vi "bats.parser.vi"(9 "data.valid":bool, 10 "data":T1={"enabled"=[FALSE, FALSE, FALSE, FALSE, FALSE, FALSE, FALSE, FALSE], "byte"=[0, 0, 0, 0, 0, 0, 0, 0]} {"byte" format="%.0x"}, 11 "reset":bool) -> (2 "Ready.for.Udp.Input":bool)   [LabVIEW 2020]
uses:
  bats.parser.state.data.ctl
  bats.parser.state.command.ctl
  <vilib>/rvi/DataTransferAndStorage/Container/XNode/niFpgaContainer.xnode
  debug/debug.type.ctl
  <vilib>/rvi/FIFO/Fifo_Resource/nirvififoEmulationWrite.vi
  data.ctl
panel:
  out "buffer.out":u64[](array[numeric]) format="%.0x"
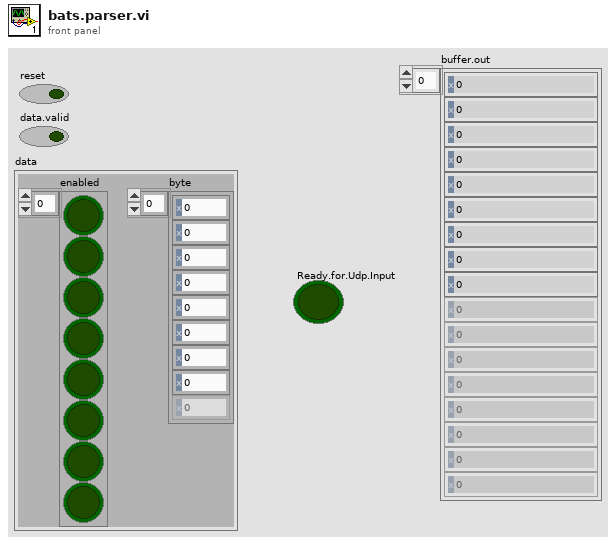
[diagram p1: front panel]
types:
  T1 = typedef "data.ctl" = cluster{"enabled":bool[], "byte":u8[]}
  T2 = typedef "bats.parser.state.command.ctl" = enum16{"Reset", "Noop", "Read.Sequenced.Unit.Header", "Read.Msg"}
  T3 = typedef "bats.parser.state.data.ctl" = cluster{"BATS.Parser.States":T2, "Saved.BATS.Parser.State":T2, "Hdr Length (U16)":u16, "MessageLength (U8)":u8, "MessageType (U8)":u8, "Time (U32)":u32, "Total Counter (U16)":u16, "Message Counter (U8)":u8, "i":u16, "Number.of.Tickers":u16, "n":u16, "msg.counter":u8, "msg.length":u8, "buffer.start":u8, "buffer.length":u8, "buffer":u64[], "Debug":T4}
  T4 = typedef "debug.type.ctl" = cluster{"Write.to.Debug":bool, "Data":u64}
  T5 = cluster{"reset":bool, "data":T1, "data.valid":bool}
  T6 = typedef "orderbook.command.ctl" = cluster{"type":T7, "side":u8, "orderId ":u64, "quantity":u32, "symbol":u64, "price":u64, "executed.qty":u32, "canceled.qty":u32, "remaining.qty":u32, "seconds":u64, "nanoseconds":u64, "Add":bool, "Edit":bool, "Remove":bool}
  T7 = typedef "orderbook.command.type.ctl" = enum8{"Time", "AddOrder", "OrderExecuted", "OrderExecutedAtPrice", "ReduceSize", "ModifyOrder", "DeleteOrder", "Get.Everything", "Get.All.Orders", "Get.Top"}
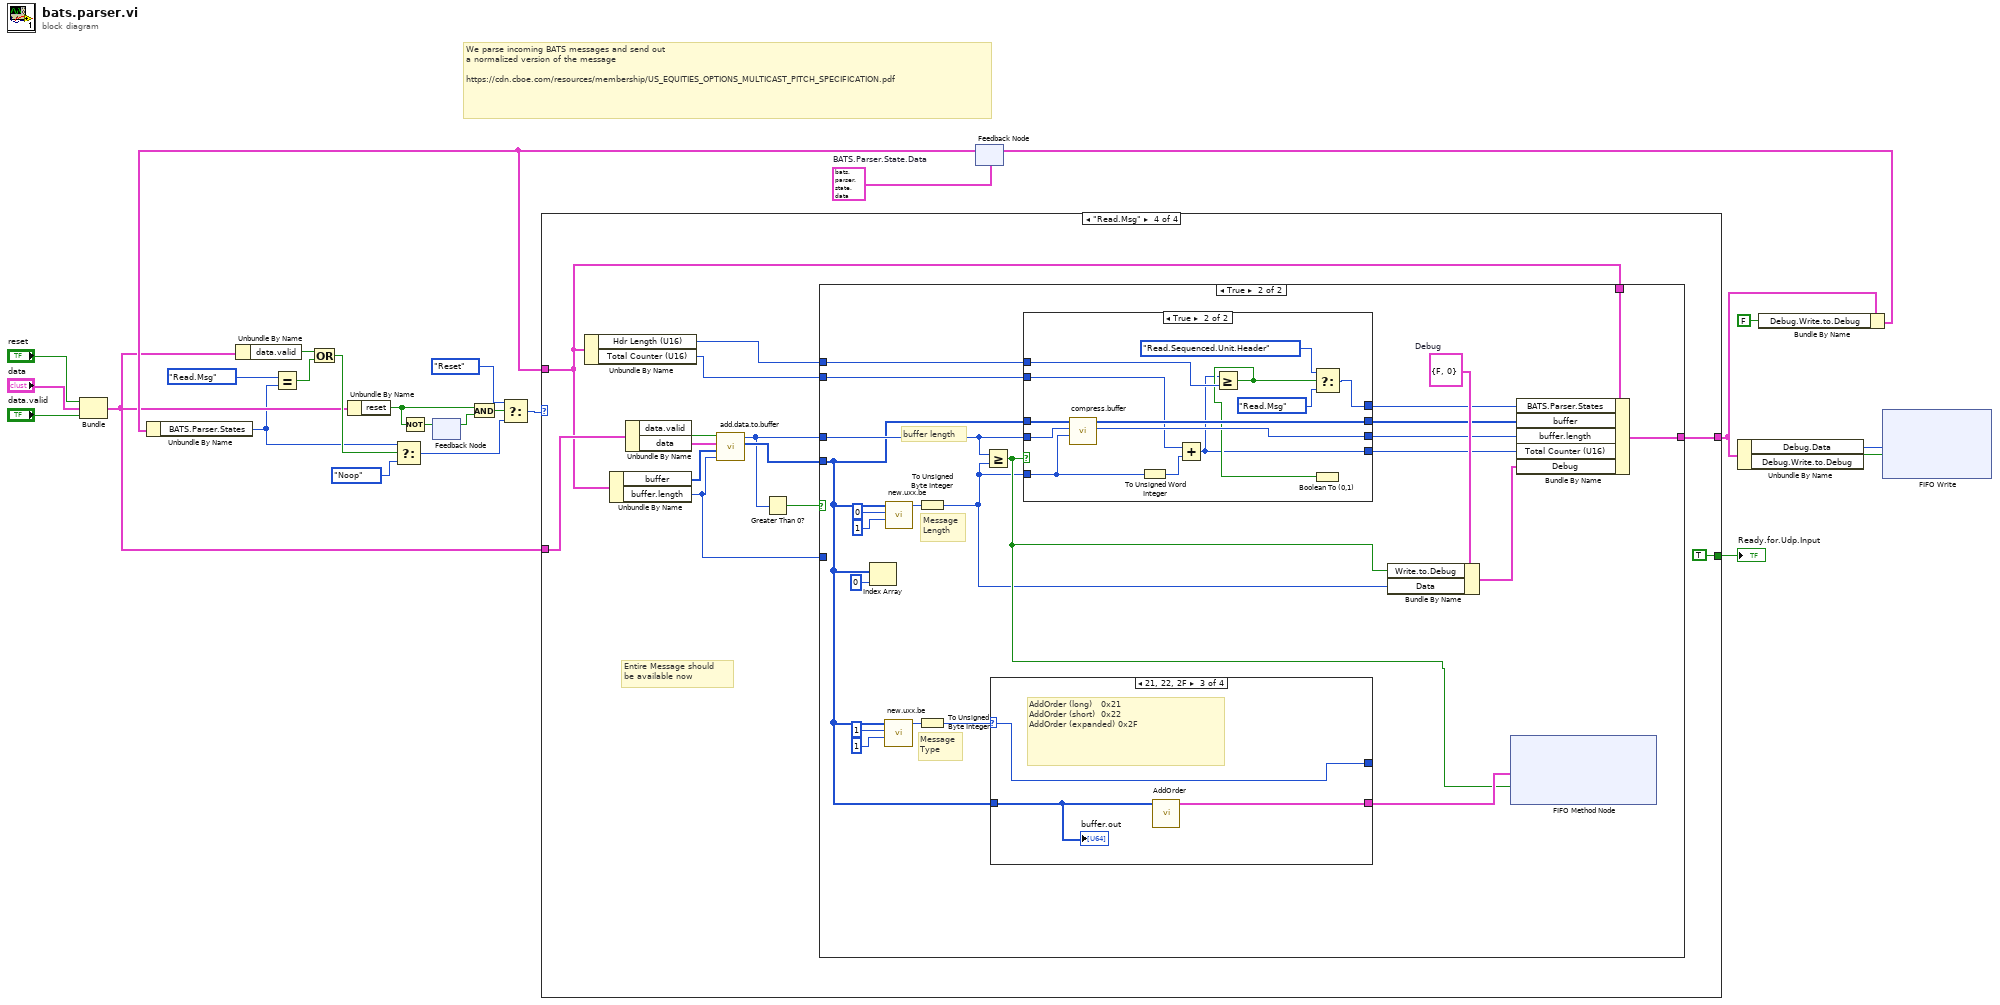
[diagram p0: block diagram]
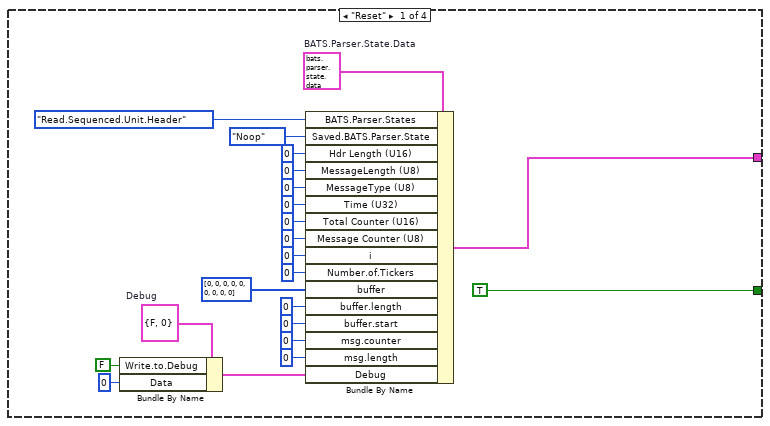
[diagram p2: hidden frame]
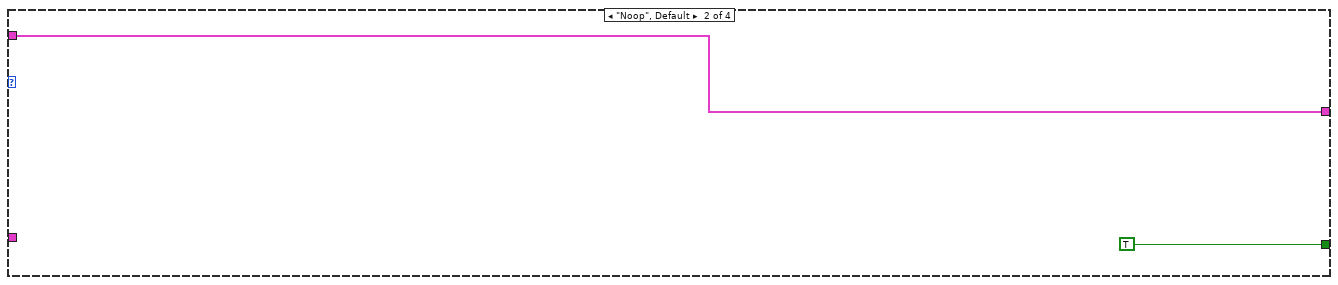
[diagram p3: hidden frame]
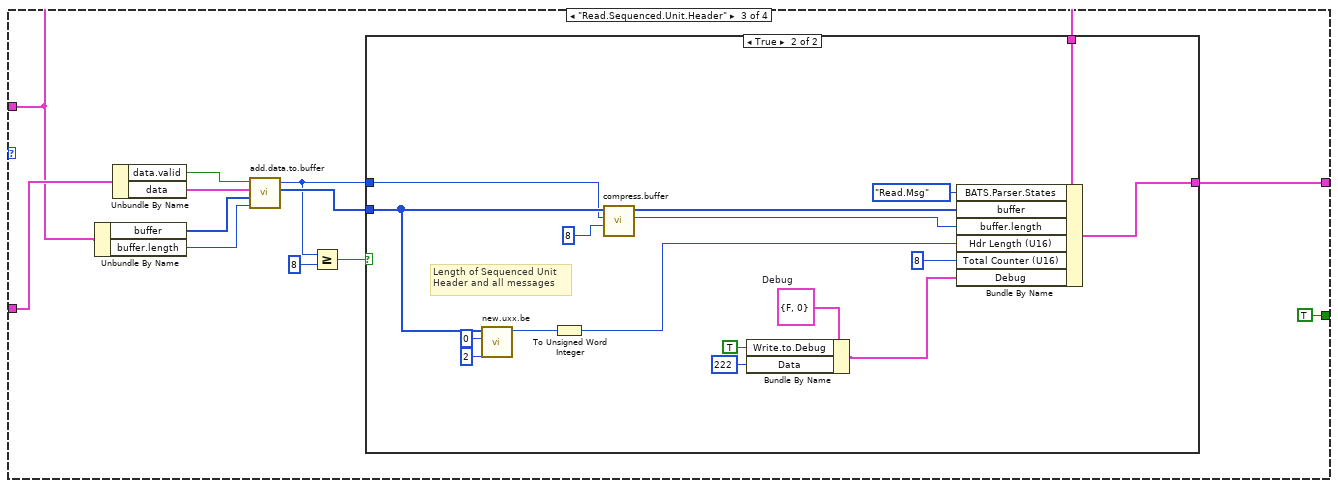
[diagram p4: hidden frame]
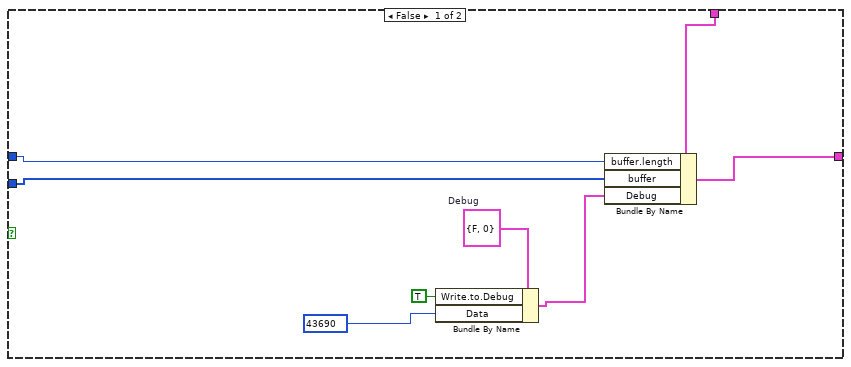
[diagram p5: hidden frame]
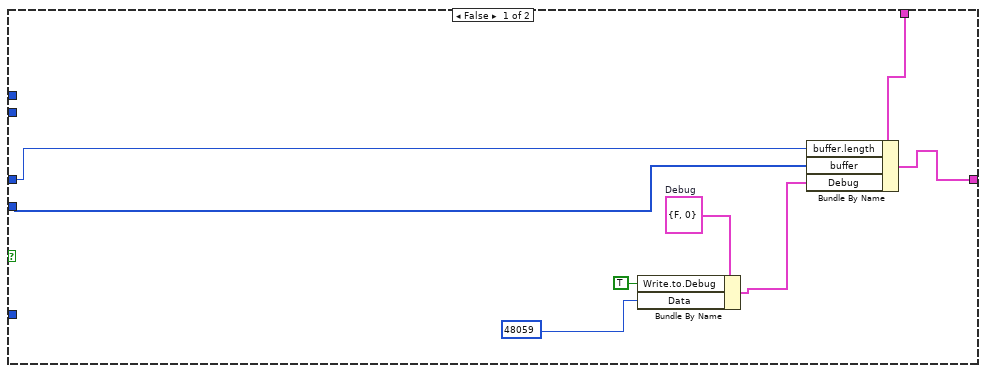
[diagram p6: hidden frame]
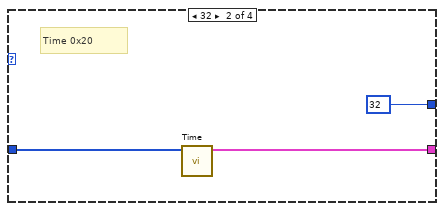
[diagram p8: hidden frame]
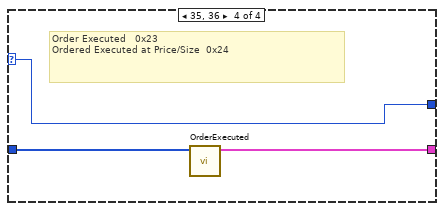
[diagram p9: hidden frame]
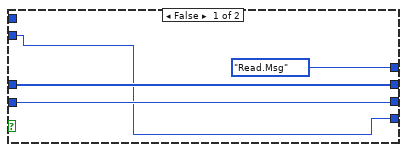
[diagram p10: hidden frame]
diagram:
  w25 = T3 {"BATS.Parser.States"=enum."Read.Sequenced.Unit.Header", "Saved.BATS.Parser.State"=enum."Reset", "Hdr Length (U16)"=0, "MessageLength (U8)"=0, "MessageType (U8)"=0, "Time (U32)"=0, "Total Counter (U16)"=0, "Message Counter (U8)"=0, "i"=0, "Number.of.Tickers"=0, "n"=0, "msg.counter"=0, "msg.length"=0, "buffer.start"=0, "buffer.length"=0, "buffer"=[0, 0, 0, 0, 0, 0, 0, 0, 0], "Debug"={"Write.to.Debug"=FALSE, "Data"=0}}  # BATS.Parser.State.Data
  # "We parse incoming BATS messages and send out\na normalized version of the message\n\nhttps://cdn.cboe.com/resources/membership/US_EQUITIES_OPTIONS_MULTICAST_PITCH_SPECIFICATION.pdf"
  n1 = Bundle("reset"="reset", "data"="data", "data.valid"="data.valid") -> (w7:T5)  [unwired: 1 in]
  n2 = Unbundle By Name(w7) -> ("data.valid"=w10:bool)
  n3 = Unbundle By Name(w7) -> ("reset"=w13:bool)
  n4 = Not(x=w13) -> (.not. x?=w16:bool)
  n5 = feedback-in #1(w16) -> ()
  n6 = feedback #1() -> (w17:bool)  [unwired: 1 in]
  n7 = And(x=w13, y=w17) -> (x .and. y?=w18:bool)
  n8 = feedback #2(w25) -> (w23:T3)
  n9 = Unbundle By Name(w23) -> ("BATS.Parser.States"=w6:T2)
  n10 = Equal?(x=bats.parser.state.command."Read.Msg" ("BATS.Parser.States"), y=w6) -> (x = y?=w19:bool)
  n11 = Compound Arithmetic op=OR(w10, w19) -> (w9:bool)
  n12 = Select(t=w6, s=w9, f=bats.parser.state.command."Noop" ("BATS.Parser.States")) -> (s? t:f=w8:T2)
  n13 = Select(t=bats.parser.state.command."Reset" ("BATS.Parser.States"), s=w18, f=w8) -> (s? t:f=w21:T2)
  n14 = case shown="\"Read.Msg\"" w21 {
    tunnel: w23 -> [_ w49 w54 w91]
    tunnel: [w46 w49 w56 w95] -> w4
    tunnel: [TRUE ("Ready for Input") TRUE ("Ready for Input") TRUE ("Ready for Input") TRUE ("Ready for Input")] -> w15
    tunnel: w7 -> [_ _ w57 w96]
    frame "Reset" {
      w31 = T4 {"Write.to.Debug"=FALSE, "Data"=0}  # Debug
      w47 = T3 {"BATS.Parser.States"=enum."Read.Sequenced.Unit.Header", "Saved.BATS.Parser.State"=enum."Reset", "Hdr Length (U16)"=0, "MessageLength (U8)"=0, "MessageType (U8)"=0, "Time (U32)"=0, "Total Counter (U16)"=0, "Message Counter (U8)"=0, "i"=0, "Number.of.Tickers"=0, "n"=0, "msg.counter"=0, "msg.length"=0, "buffer.start"=0, "buffer.length"=0, "buffer"=[0, 0, 0, 0, 0, 0, 0, 0, 0], "Debug"={"Write.to.Debug"=FALSE, "Data"=0}}  # BATS.Parser.State.Data
      n15 = Bundle By Name(cluster=w31, "Write.to.Debug"=FALSE, "Data"=u64 0) -> (w30:T4)
      n16 = Bundle By Name(cluster=w47, "BATS.Parser.States"=bats.parser.state.command."Read.Sequenced.Unit.Header", "Saved.BATS.Parser.State"=bats.parser.state.command."Noop" ("BATS.Parser.States"), "Hdr Length (U16)"=u16 0, "MessageLength (U8)"=u8 0, "MessageType (U8)"=u8 0, "Time (U32)"=u32 0, "Total Counter (U16)"=u16 0, "Message Counter (U8)"=u8 0, "i"=u16 0, "Number.of.Tickers"=u16 0, "buffer"=u64[] [0, 0, 0, 0, 0, 0, 0, 0, 0], "buffer.length"=u8 0, "buffer.start"=u8 0, "msg.counter"=u8 0, "msg.length"=u8 0, "Debug"=w30) -> (w46:T3)
    }
    frame "Noop", Default {
    }
    frame "Read.Sequenced.Unit.Header" {
      n17 = Unbundle By Name(w54) -> ("buffer"=w59:u64[], "buffer.length"=w58:u8)
      n18 = Unbundle By Name(w57) -> ("data.valid"=w60:bool, "data"=w61:T1)
      n19 = call "add.data.to.buffer.vi"("buffer.length"=w58, "buffer"=w59, "data"=w61, "data.valid"=w60) -> ("buffer.out"=w55:u64[], "buffer.length.out"=w52:u8)  [unwired: 6 in]
      n20 = Greater Or Equal?(x=w52, y=u8 8) -> (x >= y?=w53:bool)
      n21 = case shown="True" w53 {
        tunnel: [w66 w86] -> w56
        tunnel: w55 -> [w63 w81]
        tunnel: w52 -> [w64 w73]
        tunnel: w54 -> [w65 w84]
        frame False {
          w67 = T4 {"Write.to.Debug"=FALSE, "Data"=0}  # Debug
          n22 = Bundle By Name(cluster=w67, "Write.to.Debug"=TRUE, "Data"=u64 43690) -> (w69:T4)
          n23 = Bundle By Name(cluster=w65, "buffer.length"=w64, "buffer"=w63, "Debug"=w69) -> (w66:T3)
        }
        frame True {
          w77 = T4 {"Write.to.Debug"=FALSE, "Data"=0}  # Debug
          # "Length of Sequenced Unit\nHeader and all messages"
          n24 = call "new.uxx.be.vi"("buffer (U64)"=w81, "Start.Idx"=u8 0, "Length"=u8 2) -> ("Uxx.be"=w78:u64)  [unwired: 7 in]
          n25 = To Unsigned Word Integer(number=w78) -> (unsigned 16bit integer=w71:u16)
          n26 = call "compress.buffer.vi"("start.idx"=u8 8, "buffer.length"=w73, "buffer"=w81) -> ("buffer.length.out"=w72:u8, "buffer.out"=w79:u64[])  [unwired: 7 in]
          n27 = Bundle By Name(cluster=w77, "Write.to.Debug"=TRUE, "Data"=u64 222) -> (w75:T4)
          n28 = Bundle By Name(cluster=w84, "BATS.Parser.States"=bats.parser.state.command."Read.Msg", "buffer"=w79, "buffer.length"=w72, "Hdr Length (U16)"=w71, "Total Counter (U16)"=u16 8, "Debug"=w75) -> (w86:T3)
        }
      }
    }
    frame "Read.Msg" {
      # "Entire Message should \nbe available now"
      n29 = Unbundle By Name(w91) -> ("Hdr Length (U16)"=w90:u16, "Total Counter (U16)"=w89:u16)
      n30 = Unbundle By Name(w91) -> ("buffer"=w97:u64[], "buffer.length"=w88:u8)
      n31 = Unbundle By Name(w96) -> ("data.valid"=w98:bool, "data"=w99:T1)
      n32 = call "add.data.to.buffer.vi"("buffer.length"=w88, "buffer"=w97, "data"=w99, "data.valid"=w98) -> ("buffer.out"=w94:u64[], "buffer.length.out"=w93:u8)  [unwired: 6 in]
      n33 = Greater Than 0?(x=w93) -> (x > 0?=w92:bool)
      n34 = case shown="True" w92 {
        tunnel: [w106 w130] -> w95
        tunnel: w94 -> [w105 w110]
        tunnel: w93 -> [w101 w114]
        tunnel: w91 -> [w107 w129]
        tunnel: w90 -> [_ w118]
        tunnel: w89 -> [_ w117]
        tunnel: w88 -> [_ _]
        frame False {
          w102 = T4 {"Write.to.Debug"=FALSE, "Data"=0}  # Debug
          n35 = Bundle By Name(cluster=w102, "Write.to.Debug"=TRUE, "Data"=u64 48059) -> (w104:T4)
          n36 = Bundle By Name(cluster=w107, "buffer.length"=w101, "buffer"=w105, "Debug"=w104) -> (w106:T3)
        }
        frame True {
          w125 = T4 {"Write.to.Debug"=FALSE, "Data"=0}  # Debug
          # "buffer length"
          # "Message\nType"
          # "Message\nLength"
          n37 = Index Array(array=w110, index=0) -> ()  [unwired: 1 out]
          n38 = call "new.uxx.be.vi"("buffer (U64)"=w110, "Start.Idx"=u8 1, "Length"=u8 1) -> ("Uxx.be"=w123:u64)  [unwired: 7 in]
          n39 = call "new.uxx.be.vi"("buffer (U64)"=w110, "Start.Idx"=u8 0, "Length"=u8 1) -> ("Uxx.be"=w126:u64)  [unwired: 7 in]
          n40 = To Unsigned Byte Integer(number=w126) -> (unsigned 8bit integer=w108:u8)
          n41 = To Unsigned Byte Integer(number=w123) -> (unsigned 8bit integer=w113:u8)
          n42 = Greater Or Equal?(x=w114, y=w108) -> (x >= y?=w109:bool)
          n43 = case shown="21, 22, 2F" w113 {
            selector: w113 -> [w131 _ w136 w138]
            tunnel: [w131 u64 32 ("unsigned 8bit integer") w136 w138] -> _
            tunnel: [_ w134 w137 w140] -> w115
            tunnel: w110 -> [_ w133 w135 w139]
            frame 0, Default {
              # "Other/Unsupported"
            }
            frame 32 {
              # "Time 0x20"
              n44 = call "Time.vi"("buffer.in"=w133) -> ("OrderBook.Command"=w134:T6)  [unwired: 10 in]
            }
            frame 33, 34, 47 {
              # "AddOrder (long)   0x21\nAddOrder (short)  0x22\nAddOrder (expanded) 0x2F"
              n45 = call "AddOrder.vi"("buffer.in"=w135) -> ("OrderBook.Command"=w137:T6)  [unwired: 10 in]
              "buffer.out" <- w135
            }
            frame 35, 36 {
              # "Order Executed   0x23\nOrdered Executed at Price/Size  0x24"
              n46 = call "OrderExecuted.vi"("buffer.in"=w139) -> ("OrderBook.Command"=w140:T6)  [unwired: 10 in]
            }
          }
          n47 = case shown="True" w109 {
            tunnel: [w143 w154] -> w121
            tunnel: [w144 w157] -> w122
            tunnel: w114 -> [w143 w155]
            tunnel: w110 -> [w144 w156]
            tunnel: w108 -> [_ w153]
            tunnel: [bats.parser.state.command."Read.Msg" ("BATS.Parser.States") w148] -> w120
            tunnel: [w141 w145] -> w119
            tunnel: w118 -> [_ w150]
            tunnel: w117 -> [w141 w151]
            frame False {
            }
            frame True {
              n48 = call "compress.buffer.vi"("start.idx"=w153, "buffer.length"=w155, "buffer"=w156) -> ("buffer.length.out"=w154:u8, "buffer.out"=w157:u64[])  [unwired: 7 in]
              n49 = To Unsigned Word Integer(number=w153) -> (unsigned 16bit integer=w152:u16)
              n50 = Add(x=w151, y=w152) -> (x+y=w145:u16)
              n51 = Greater Or Equal?(x=w145, y=w150) -> (x >= y?=w146:bool)
              n52 = Boolean To (0,1)(Boolean=w146) -> ()  [unwired: 1 out]
              n53 = Select(t=bats.parser.state.command."Read.Sequenced.Unit.Header", s=w146, f=bats.parser.state.command."Read.Msg" ("BATS.Parser.States")) -> (s? t:f=w148:T2)
            }
          }
          n54 = Bundle By Name(cluster=w125, "Write.to.Debug"=w109, "Data"=w108) -> (w116:T4)
          n55 = xnode ("FIFO Method Node")("Element"=w115, "Input Valid"=w109) -> ()  [unwired: 1 in, 2 out]
          n56 = Bundle By Name(cluster=w129, "BATS.Parser.States"=w120, "buffer"=w122, "buffer.length"=w121, "Total Counter (U16)"=w119, "Debug"=w116) -> (w130:T3)
        }
      }
    }
  }
  "Ready.for.Udp.Input" <- w15
  n57 = Unbundle By Name(w4) -> ("Debug.Data"=w3:u64, "Debug.Write.to.Debug"=w1:bool)
  n58 = Bundle By Name(cluster=w4, "Debug.Write.to.Debug"=FALSE) -> (w12:T3)
  n59 = feedback-in #2(w12) -> ()
  n60 = xnode ("FIFO Write")("Element"=w3, "Input Valid"=w1) -> ()  [unwired: 1 in, 2 out]
